vi "Handling Common User Interface Events.vi"() -> ()   [LabVIEW 2023]
doc: "Tracks which user interface events are happening with the Event Structure. Run the VI and follow the instructions on the front panel. The Captured Events string displays which events have occurred."
panel:
  in  "Stop":bool
  out "Captured Events":string
  in  "Vertical Pointer Slide":dbl(slide) scale=0.0..4.0
  in  "Play Button":bool
  in  "String Control":string
  # "Overview: Demonstrates the use of the Event Structure to handle common user interface events.\nInstructions:\n1. Run the VI.\n2. Type values in the String Control and observe the Key Down and Key Repeat events that occur.\n3. Change the value of the Play Button and the Vertical Pointer Slide and observe the Value Change events that occur.\n4. Select items in the VI menubar and observe the Menu Selection events that occur.\n5. Click Stop to stop the VI."
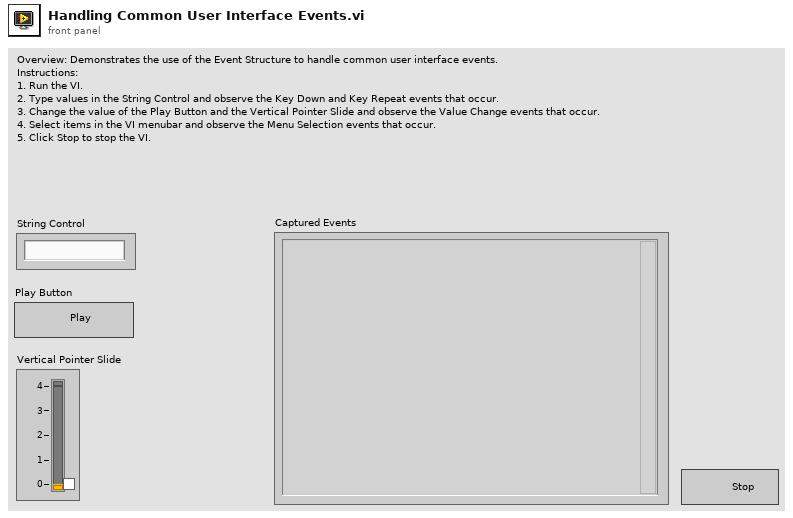
[diagram p1: front panel]
types:
  T1 = typedef "lveventtype.ctl" = enum32{"Null", "Timeout", "Annotation Menu Selection", "Annotation Menu Selection?", "App Instance Close", "App Instance Close?", "Autoscale Range Change", "Bookmark Info Change", "Cell Edit", "Cell Edit?", "Cursor Grab", "Cursor Grab?", "Cursor Menu Selection", "Cursor Menu Selection?", "Cursor Move", "Cursor Release", "Data Change", "Direction Change", "Display State Change", "Drag Ended", "Drag Enter", "Drag Leave", "Drag Over", "Drag Source Update", "Drag Starting", "Drag Starting?", "Drop", "Exec State Change", "Key Down", "Key Down?", "Key Repeat", "Key Repeat?", "Key Up", "Listbox Double Click", "Menu Activation?", "Menu Selection (App)", "Menu Selection? (App)", "Menu Selection (User)", "Mouse Down", "Mouse Down?", "Mouse Enter", "Mouse Leave", "Mouse Move", "Mouse Up", "Mouse Wheel", "NI Security User Change (App)", "Pane Size", "Panel Close", "Panel Close?", "Panel Resize", "Plot Attribute Change", "Scale Range Change", "Shortcut Menu Activation?", "Shortcut Menu Selection (App)", "Shortcut Menu Selection? (App)", "Shortcut Menu Selection (User)", "Tree Double Click", "Tree Drag", "Tree Drag?", "Tree Drop", "Tree Drop?", "Tree Item Close", "Tree Item Close?", "Tree Item Open", "Tree Item Open?", "User Event", "Value Change"}
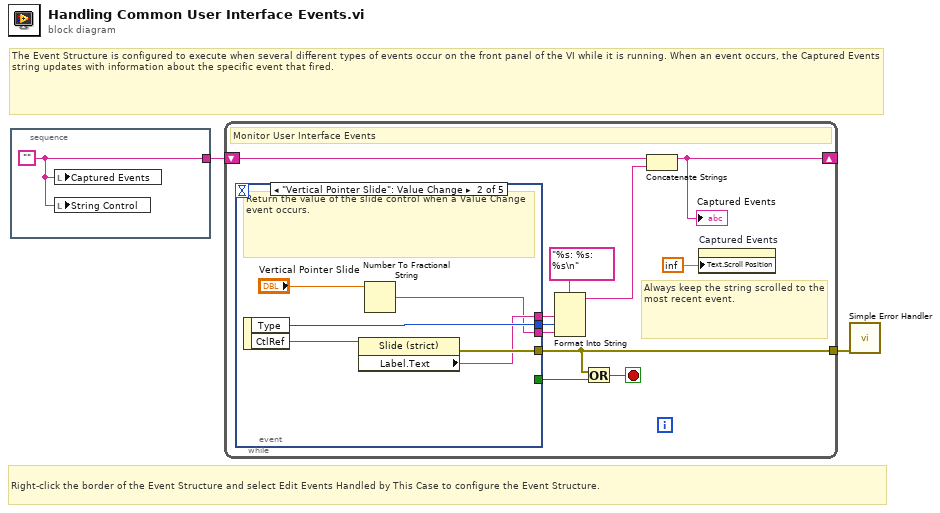
[diagram p0: block diagram]
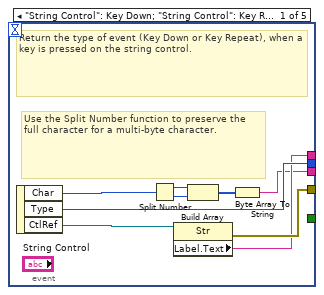
[diagram p2: hidden frame]
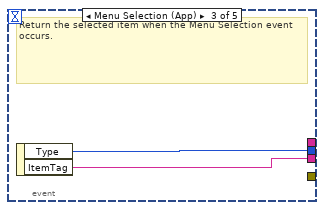
[diagram p3: hidden frame]
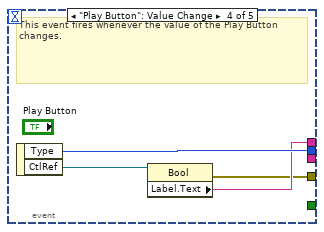
[diagram p4: hidden frame]
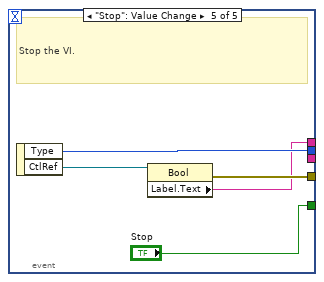
[diagram p5: hidden frame]
diagram:
  # "Right-click the border of the Event Structure and select Edit Events Handled by This Case to configure the Event Structure."
  # "The Event Structure is configured to execute when several different types of events occur on the front panel of the VI while it is running. When an event occurs, the Captured Events string updates with information about the specific event that fired."
  n1 = stacked-sequence {
    tunnel: [w3] -> w2
    frame #0 {
      w3 = ""
      n2 = local write "Captured Events"(w3) -> ()
      n3 = local write "String Control"(w3) -> ()
    }
  }
  n4 = while {
    shift-right: [w14] -> _
    shift-left: w2 -> [w13]
    tunnel: [w10] -> w1
    stop <- w11 stop-if-true
    # "Always keep the string scrolled to the most recent event."
    # "Monitor User Interface Events"
    n5 = event shown="[1] \"Vertical Pointer Slide\": Value Change" {
      selector: _ -> [_ _ _ _ _]
      dyn-events: _ -> [_ _ _ _ _]
      timeout: _ -> [_ _ _ _ _]
      tunnel: [_ _ _ _ "Stop"] -> w12
      tunnel: [w21 w28 _ w33 w39] -> w10
      tunnel: [w20 w27 w31 w35 w38] -> w7
      tunnel: [w19 w26 _ w34 w37] -> w6
      tunnel: [w18 w25 w30 _ _] -> w4
      event "String Control": Key Down; "String Control": Key Repeat {
        # "Use the Split Number function to preserve the full character for a multi-byte character."
        # "Return the type of event (Key Down or Key Repeat), when a key is pressed on the string control."
        n6 = event-data() -> ("Char"=w17:i16, "Type"=w20:T1, "CtlRef"=w22:refnum<vi>)  [unwired: 1 out]
        n7 = Split Number(x=w17) -> (hi(x)=w16:u8, lo(x)=w15:u8)
        n8 = property class="Str"(reference=w22) -> (error out=w21:errorcluster, "Label.Text"=w19:string)  [unwired: 1 in, 1 out]
        n9 = Build Array(w16, w15) -> (w23:u8[])
        n10 = Byte Array To String(unsigned byte array=w23) -> (string=w18:string)
      }
      event "Vertical Pointer Slide": Value Change {
        # "Return the value of the slide control when a Value Change event occurs."
        n11 = event-data() -> ("Type"=w27:T1, "CtlRef"=w29:refnum<vi>)  [unwired: 1 out]
        n12 = property class="Slide (strict)"(reference=w29) -> (error out=w28:errorcluster, "Label.Text"=w26:string)  [unwired: 1 in, 1 out]
        n13 = Number To Fractional String(number="Vertical Pointer Slide") -> (F-format string=w25:string)  [unwired: 3 in]
      }
      event Menu Selection (App) {
        # "Return the selected item when the Menu Selection event occurs."
        n14 = event-data() -> ("Type"=w31:T1, "ItemTag"=w30:string)  [unwired: 1 out]
      }
      event "Play Button": Value Change {
        # "This event fires whenever the value of the Play Button changes."
        n15 = event-data() -> ("Type"=w35:T1, "CtlRef"=w32:refnum<vi>)  [unwired: 1 out]
        n16 = property class="Bool"(reference=w32) -> (error out=w33:errorcluster, "Label.Text"=w34:string)  [unwired: 1 in, 1 out]
      }
      event "Stop": Value Change {
        # "Stop the VI."
        n17 = event-data() -> ("Type"=w38:T1, "CtlRef"=w36:refnum<vi>)  [unwired: 1 out]
        n18 = property class="Bool"(reference=w36) -> (error out=w39:errorcluster, "Label.Text"=w37:string)  [unwired: 1 in, 1 out]
      }
    }
    n19 = Format Into String(format string="%s: %s: %s\n", w6, w7, w4) -> (resulting string=w5:string)  [unwired: 2 in, 1 out]
    n20 = Or(x=w10, y=w12) -> (x .or. y?=w11:bool)
    n21 = Concatenate Strings(w13, w5) -> (w14:string)
    "Captured Events" <- w14
    n22 = property on="Captured Events" class="Str"("Text.Scroll Position"=inf) -> ()  [unwired: 2 in, 2 out]
  }
  n23 = call <vilib>:"Simple Error Handler.vi"("error in (no error)"=w1) -> ()  [unwired: 4 in, 5 out]
